vi "GetRoutingParameter.vi"(11 "Parameters":T1[](array[typedef])) -> (2 "Found":bool, 3 "RoutingParameter":T1)   [LabVIEW 2017, in "MessageGen.lvlib"]
uses:
  <vilib>/addons/InsightCM/MessageBus/CodeGen/MessageGen.lvlib
  <vilib>/addons/InsightCM/MessageBus/CodeGen/controls/Parameter.ctl
  <vilib>/addons/InsightCM/MessageBus/CodeGen/controls/ParameterType.ctl
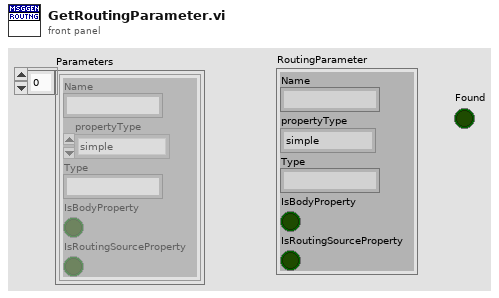
[diagram p1: front panel]
types:
  T1 = typedef "MessageGen.lvlib/Parameter.ctl" = cluster{"Name":string, "propertyType":T2, "Type":string, "IsBodyProperty":bool, "IsRoutingSourceProperty":bool}
  T2 = typedef "MessageGen.lvlib/ParameterType.ctl" = enum16{"simple", "bytearray", "dateTime", "list", "map", "object"}
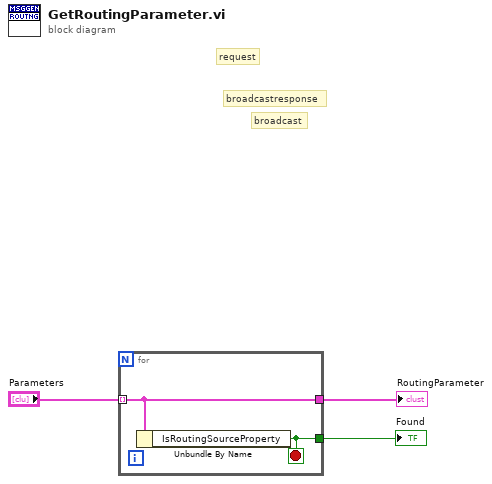
[diagram p0: block diagram]
diagram:
  # "broadcast"
  # "broadcastresponse"
  # "request"
  n1 = for {
    tunnel: "Parameters" -> [w5] mode=indexing
    tunnel: [w5] -> w1
    tunnel: [w4] -> w2
    stop <- w4 stop-if-true
    n2 = Unbundle By Name(w5) -> ("IsRoutingSourceProperty"=w4:bool)
  }
  "Found" <- w2
  "RoutingParameter" <- w1
